vi "Play Path.vi"(6 "Reset Gyro":bool, 8 "Commands":cluster{"Time (s)":dbl, T1, bool}[](array[cluster]), 9 "Angles":dbl[](array[numeric]), 10 "Velocity":dbl[](array[numeric]), 11 "Booleans":T3) -> ()   [LabVIEW 2019]
uses:
  <vilib>/Rock Robotics/WPI/Framework/Command Status Info.ctl
  <vilib>/Rock Robotics/WPI/Framework/Completion Status.ctl
  <vilib>/Rock Robotics/WPI/Framework/Completion Notifier.ctl
  Bordeaux/bordeaux-pathinator/Bordeaux/Command Stuff/Single Cmd Info.ctl
  <vilib>/picture/picture.llb/imagedata.ctl
  Implementation/Drivebase Setpoints.ctl
  Implementation/Drivebase Operations.ctl
panel:
  in  "Description":string
  out "Command Info Out":T4
  in  "Command Info In":T4
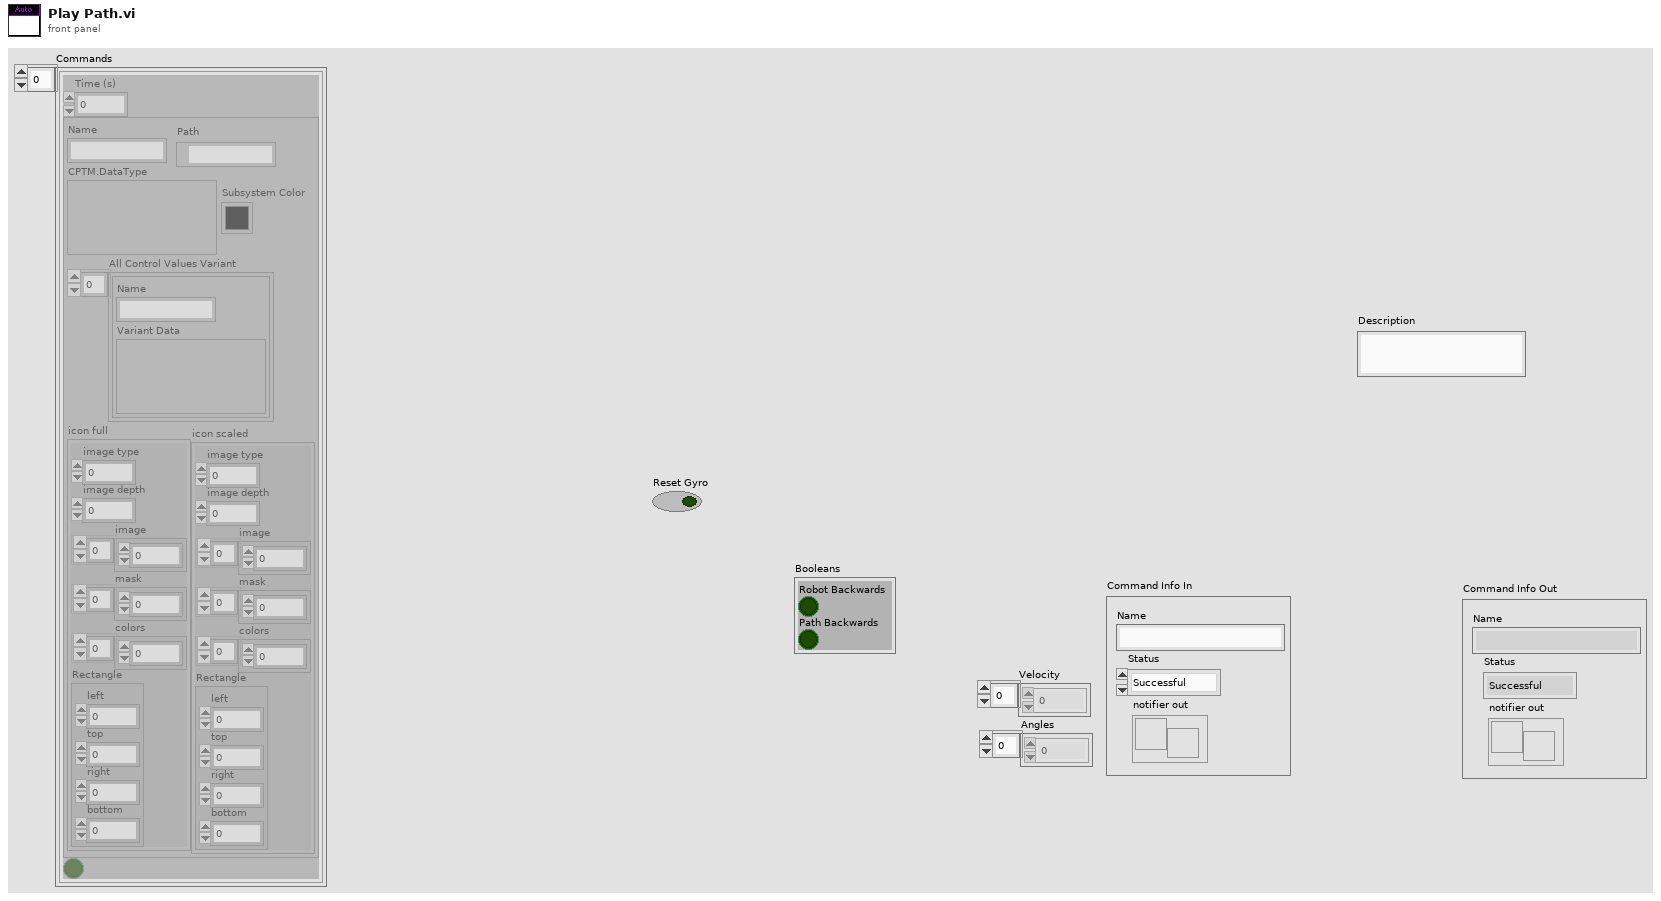
[diagram p1: front panel]
types:
  T1 = typedef "Single Cmd Info.ctl" = cluster{"Name":string, "CPTM.DataType":variant, "All Control Values Variant":cluster{"Name":string, "Variant Data":variant}[], "icon full":T2, "icon scaled":T2, "Path":path, "Subsystem Color":u32}
  T2 = typedef "imagedata.ctl" = cluster{"image type":i32, "image depth":i32, "image":u8[], "mask":u8[], "colors":u32[], "Rectangle":cluster{"left":i16, "top":i16, "right":i16, "bottom":i16}}
  T3 = cluster{"Robot Backwards":bool, "Path Backwards":bool}
  T4 = typedef "Command Status Info.ctl" = cluster{"Name":string, "Status":T5, "notifier out":T6}
  T5 = typedef "Completion Status.ctl" = enum16{"Successful", "Aborted", "Incomplete"}
  T6 = typedef "Completion Notifier.ctl" = refnum<notifier>
  T7 = typedef "Drivebase Setpoints.ctl" = cluster{"Operation":T8, "Left Setpoint":dbl, "Right Setpoint":dbl, "Velocity":dbl[], "Angles":dbl[], "Reset Gyro":bool, "Booleans":cluster{"Robot Backwards":bool, "Path Backwards":bool}, "Commands":cluster{"Time (s)":dbl, T1, bool}[]}
  T8 = typedef "Drivebase Operations.ctl" = enum16{"Reserve", "Read Current", "Immediate", "Pathinator"}
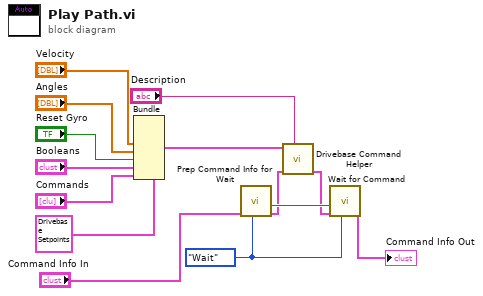
[diagram p0: block diagram]
diagram:
  w2 = enum16{"Start", "Wait"}."Wait" ("Synchronication")
  n1 = Bundle(cluster=T7 {"Operation"=enum."Pathinator", "Left Setpoint"=0.0, "Right Setpoint"=0.0, "Velocity"=[], "Angles"=[], "Reset Gyro"=FALSE, "Booleans"={"Robot Backwards"=FALSE, "Path Backwards"=FALSE}, "Commands"=[]} ("SubSystem Data"), "Velocity"="Velocity", "Angles"="Angles", "Reset Gyro"="Reset Gyro", "Booleans"="Booleans", "Commands"="Commands") -> (w12:T7)  [unwired: 3 in]
  n2 = call <vilib>:"Prep Command Info for Wait.vi"("Synchronication"=w2, "Command Info"="Command Info In") -> ("Command Info"=w7:T4, "Allocated"=w9:bool)  [unwired: 8 in]
  n3 = call "Drivebase Command Helper.vi"("Description"="Description", "Command Info In"=w7, "SubSystem Data"=w12) -> ("Command Info Out"=w8:T4)  [unwired: 6 in, 2 out]
  n4 = call <vilib>:"Wait for Command.vi"("Synchronication"=w2, "Command Info in"=w8, "Allocated"=w9) -> ("Command Info out"=→"Command Info Out":T4)  [unwired: 8 in]
